vi "Generator.Create AO DC waveforms.vi"(8 "error in (no error)":errorcluster, 9 "sweep state":T1=enum."sweep", 11 "Generator in":refnum<class "Generator.lvclass">) -> (0 "error out":errorcluster, 2 "AO Array":waveform(dbl)[](array[waveform]), 3 "Generator out":refnum<class "Generator.lvclass">)   [LabVIEW 2019, in "Generator.lvclass"]
uses:
  Instrument.DAQ/Typedefs/Sweep.State--enum.ctl
  Generator.lvclass
  Instrument.DAQ/Instrument.DAQ.lvclass
  C:/Program Files (x86)/National Instruments/LabVIEW 2019/vi.lib/JKI/JKI SMO/SMO/SMO.lvclass
panel:
  in  "Tab Control":enum32{"Page 1", "Graphs"}(tab)
  out "Waveform Graph":waveform(dbl)[](graph)
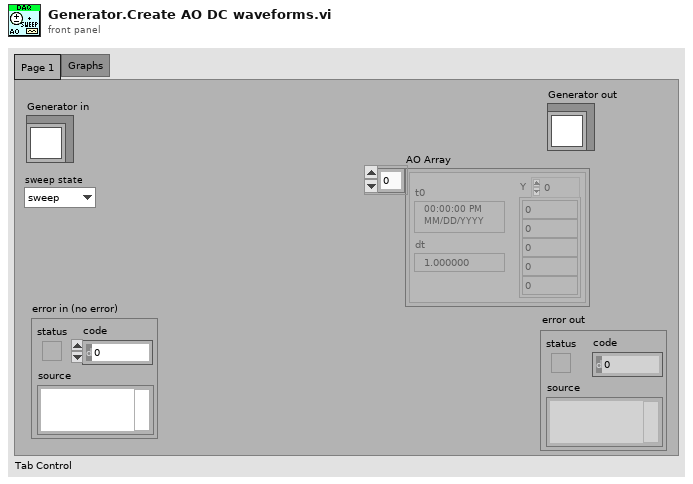
[diagram p1: front panel]
types:
  T1 = typedef "Instrument.Lockin.lvlib/Instrument.DAQ.lvclass/Sweep.State--enum.ctl" = enum16{"idle", "initialize", "wait", "sweep", "stop"}
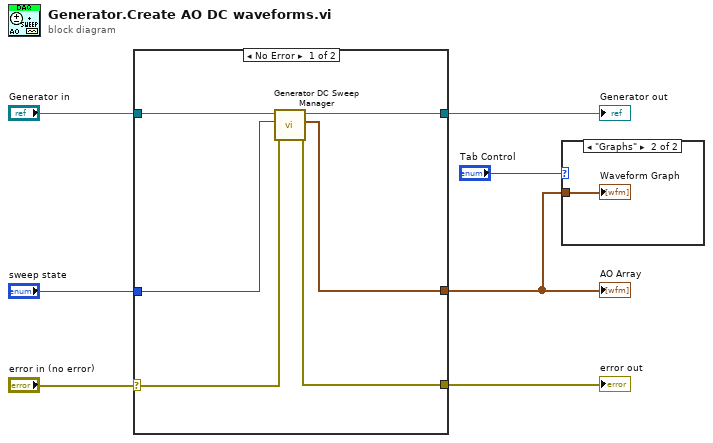
[diagram p0: block diagram]
diagram:
  n1 = case shown="No Error" "error in (no error)" {
    selector: "error in (no error)" -> [w8 w15]
    tunnel: "sweep state" -> [w13 _]
    tunnel: "Generator in" -> [w12 w14]
    tunnel: [w11 w14] -> w5
    tunnel: [w10 w15] -> w4
    tunnel: [w9 _] -> w3
    frame No Error {
      n2 = call "Generator DC Sweep Manager.vi"("error in (no error)"=w8, "sweep state"=w13, "Instrument.DAQ in"=w12) -> ("error out"=w10:errorcluster, "Waveform []"=w9:waveform(dbl)[], "Instrument.DAQ out"=w11:refnum<class "Instrument.DAQ.lvclass">)  [unwired: 6 in]
    }
    frame Error {
    }
  }
  "AO Array" <- w3
  "error out" <- w4
  "Generator out" <- w5
  n3 = case shown="\"Graphs\"" "Tab Control" {
    tunnel: w3 -> [_ w16]
    frame Default {
    }
    frame "Graphs" {
      "Waveform Graph" <- w16
    }
  }
